vi "CreateProduct.vi"(8 "error in (no error)":errorcluster, 11 "ProductB_Factory in":refnum<class "ProductB_Factory.lvclass">) -> (0 "error out":errorcluster, 2 "Product.lvclass":refnum<class "Product.lvclass">, 3 "ProductB_Factory out":refnum<class "ProductB_Factory.lvclass">)   [LabVIEW 2017, in "ProductB_Factory.lvclass"]
uses:
  ProductB_Factory.lvclass
  Product Class/Product/Product.lvclass
  Product Class/ProductA/ProductB.lvclass
  C:/Users/fflores/Desktop/LabIVEW OOP Design Patterns/Factory Method Pattern/Product Class/Product/Product.lvclass
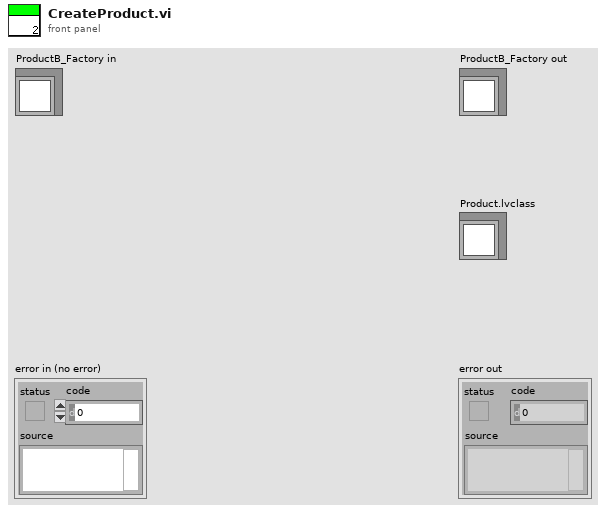
[diagram p1: front panel]
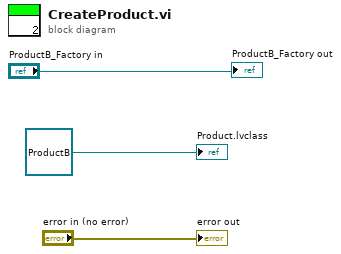
[diagram p0: block diagram]
diagram:
  "error out" <- "error in (no error)"
  "ProductB_Factory out" <- "ProductB_Factory in"
  "Product.lvclass" <- refnum<class "ProductB.lvclass"> refnum ("ProductB.lvclass")
